vi "Guia1_7n.vi"() -> ()   [LabVIEW 2016]
uses:
  <vilib>/sound2/lvsound2.llb/Sound Data Format.ctl
  <vilib>/sound2/lvsound2.llb/Sampling Mode.ctl
  <vilib>/sound2/lvsound2.llb/Sound Output Write (DBL).vi
  <vilib>/measure/NI_MABase.lvlib
panel:
  in  "Amplitud 2":dbl(knob) scale=0.0..100.0
  in  "Frecuencia  2":dbl(knob) scale=0.0..100.0
  in  "Amplitud":dbl(knob) scale=0.0..100.0
  in  "Frecuencia":dbl(knob) scale=0.0..100.0
  out "Waveform Graph":waveform(dbl)[](graph)
  in  "number of samples/ch":i32=100000
  in  "stop":bool
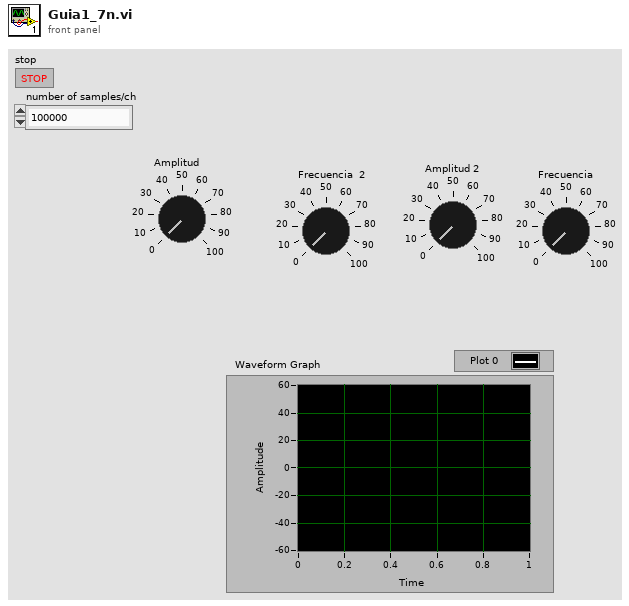
[diagram p1: front panel]
types:
  T1 = typedef "Sampling Mode.ctl" = i32
  T2 = typedef "Sound Data Format.ctl" = cluster{"sample rate (S/s)":dbl, "number of channels":i32, "bits per sample":i32}
  T3 = typedef "Sound Output Task ID.ctl" = u32
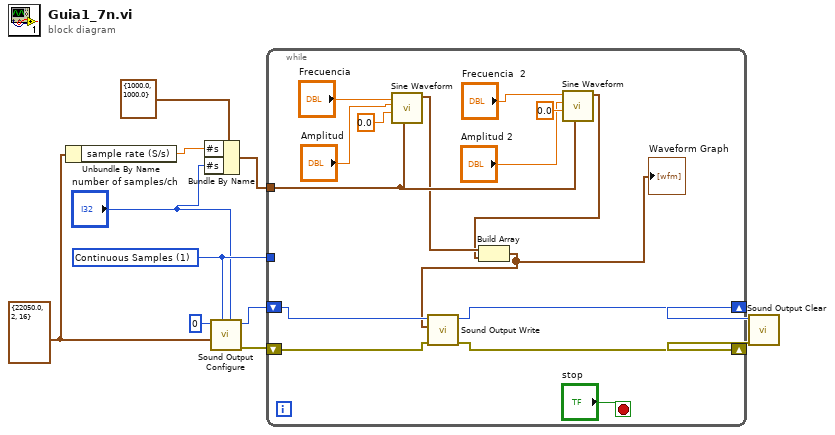
[diagram p0: block diagram]
diagram:
  w6 = T1 1 items=["Finite Samples", "Continuous Samples"] ("sample mode")
  w5 = T2 {"sample rate (S/s)"=22050.0, "number of channels"=2, "bits per sample"=16} ("sound format")
  n1 = Unbundle By Name(w5) -> ("sample rate (S/s)"=w3:dbl)
  n2 = Bundle By Name(cluster=cluster{"#s":dbl, "Fs":dbl} {"#s"=1000.0, "Fs"=1000.0} ("sampling info"), "#s"=w3, "#s"="number of samples/ch") -> (w1:cluster{"#s":dbl, "Fs":dbl})
  n3 = call <vilib>:"Sound Output Configure.vi"("number of samples/ch"="number of samples/ch", "sample mode"=w6, "sound format"=w5, "device ID"=u32 0) -> ("error out"=w11:errorcluster, "task ID"=w10:T3)  [unwired: 6 in]
  n4 = while {
    shift-right: [w23] -> w8
    shift-left: w11 -> [w24]
    shift-right: [w22] -> w9
    shift-left: w10 -> [w25]
    tunnel: w6 -> [_]
    tunnel: w1 -> [w15]
    stop <- "stop" stop-if-true
    n5 = call <vilib>:"Sine Waveform.vi"("sampling info"=w15, "phase"=0.0, "amplitude"="Amplitud", "frequency"="Frecuencia") -> ("signal out"=w14:waveform(dbl))  [unwired: 6 in, 1 out]
    n6 = call <vilib>:"Sine Waveform.vi"("sampling info"=w15, "phase"=0.0, "amplitude"="Amplitud 2", "frequency"="Frecuencia  2") -> ("signal out"=w13:waveform(dbl))  [unwired: 6 in, 1 out]
    n7 = Build Array(w14, w13) -> (w12:waveform(dbl)[])
    "Waveform Graph" <- w12
    n8 = call-poly <vilib>:"Sound Output Write.vi"("error in (no error)"=w24, "data"=w12, "task ID"=w25) -> ("error out"=w23:errorcluster, "task ID out"=w22:T3)  [unwired: 7 in]
  }
  n9 = call <vilib>:"Sound Output Clear.vi"("error in (no error)"=w8, "task ID"=w9) -> ()  [unwired: 9 in, 1 out]
